vi "Calculate Viscocity.vi"(8 "error in":errorcluster, 11 "Air in":refnum<class "Air.lvclass">) -> (0 "error out":errorcluster, 2 "mu":dbl, 3 "Air out":refnum<class "Air.lvclass">)   [LabVIEW 2013, in "Air.lvclass"]
uses:
  Air.lvclass
  Gas Properties.lvclass/Gas Properties.ctl
  Accessors/Read T (K).vi
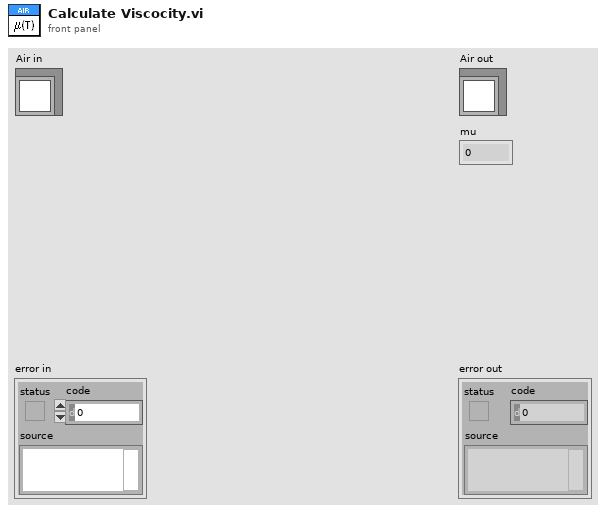
[diagram p1: front panel]
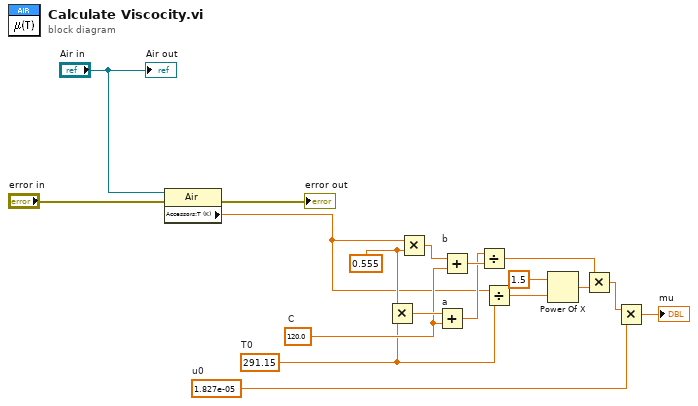
[diagram p0: block diagram]
diagram:
  w10 = 0.555 ("y")
  w7 = 1.827e-05  # u0
  w6 = 291.15  # T0
  w8 = 120.0  # C
  n1 = property class="Air"(reference="Air in", error in="error in") -> (error out=→"error out":errorcluster, "Accessors:T (K)"=w3:dbl)  [unwired: 1 out]
  n2 = Multiply(x=w10, y=w6) -> (x*y=w9:dbl)
  n3 = Multiply(x=w3, y=w10) -> (x*y=w11:dbl)
  n4 = Add "a"(x=w9, y=w8) -> (x+y=w15:dbl)
  n5 = Add "b"(x=w11, y=w8) -> (x+y=w16:dbl)
  n6 = Divide(x=w15, y=w16) -> (x/y=w14:dbl)
  n7 = Divide(x=w3, y=w6) -> (x/y=w18:dbl)
  n8 = Power Of X(1:w18, 2:1.5 ("y")) -> (0:w13:dbl)
  n9 = Multiply(x=w14, y=w13) -> (x*y=w12:dbl)
  n10 = Multiply(x=w12, y=w7) -> (x*y=→"mu":dbl)
  "Air out" <- "Air in"
